vi "总磷通讯.vi"() -> ()   [LabVIEW 2016, in "斯坦道总磷.lvlib"]
uses:
  <vilib>/NI/Modbus Library/API/Wrapper/Create TCP Slave.vi
  <vilib>/Utility/config.llb/Write Key (Boolean).vi
  <vilib>/Utility/config.llb/Write Key (String).vi
  <vilib>/Plasmionique/MB Master/MB_Master/MB_Master.lvclass
  <vilib>/NI/Modbus Library/API/slave/Modbus Slave.lvclass
  <vilib>/Utility/config.llb/NI_LVConfig.lvlib
  <vilib>/Plasmionique/MB Master/MB Master.lvlib
  <vilib>/NI/Modbus Library/API/Wrapper/API Main.lvlib
panel:
  out "总氮测量数据区":u16[](array[numeric])
  out "总氮状态告警区":u16[](array[numeric])
  out "总磷状态告警区":u16[](array[numeric])
  out "总磷测量数据区":u16[](array[numeric])
  out "序列号":string
  out "状态告警区":T1
  out "测量数据区":T2 {"单位" items=["ug/L", "mg/L", "ppm", "mg/m3", "cm", "ppb", "ug/m3", "%", "nmol/mol", "umol/mol", "MPN/L", "MPN/100ml", "ng/m3", "NTU", "无量纲", "ms/cm", "us/cm", "℃", "mV", "万个/L"]}
  out "status":bool
  out "关键参数区":T3
  in  "读关键参数区":bool
  in  "读状态告警区":bool
  in  "读测量数据区":bool
  in  "站号":u16(ring) items=["总磷"=1, "氨氮"=3]
  in  "停止":bool
  in  "启动":bool
  in  "控制命令":u16(ring) items=["启动测量"=1, "标样核查"=2, "零点核查"=3, "跨度核查"=4, "空白测试"=5, "平行样测试"=6, "加标回收"=7, "空白校准"=8, "标样校准"=9, "初始化（清洗）"=10, "停止测试"=11, "仪器重启"=12, "校时"=13, "模式设置"=14, "测量间隔设置"=15]
  in  "控制命令参数":u16[](array[numeric]) format="%04xH"
  in  "VISA Resource":refnum<visa-resource-name>
  in  "启用模块":bool
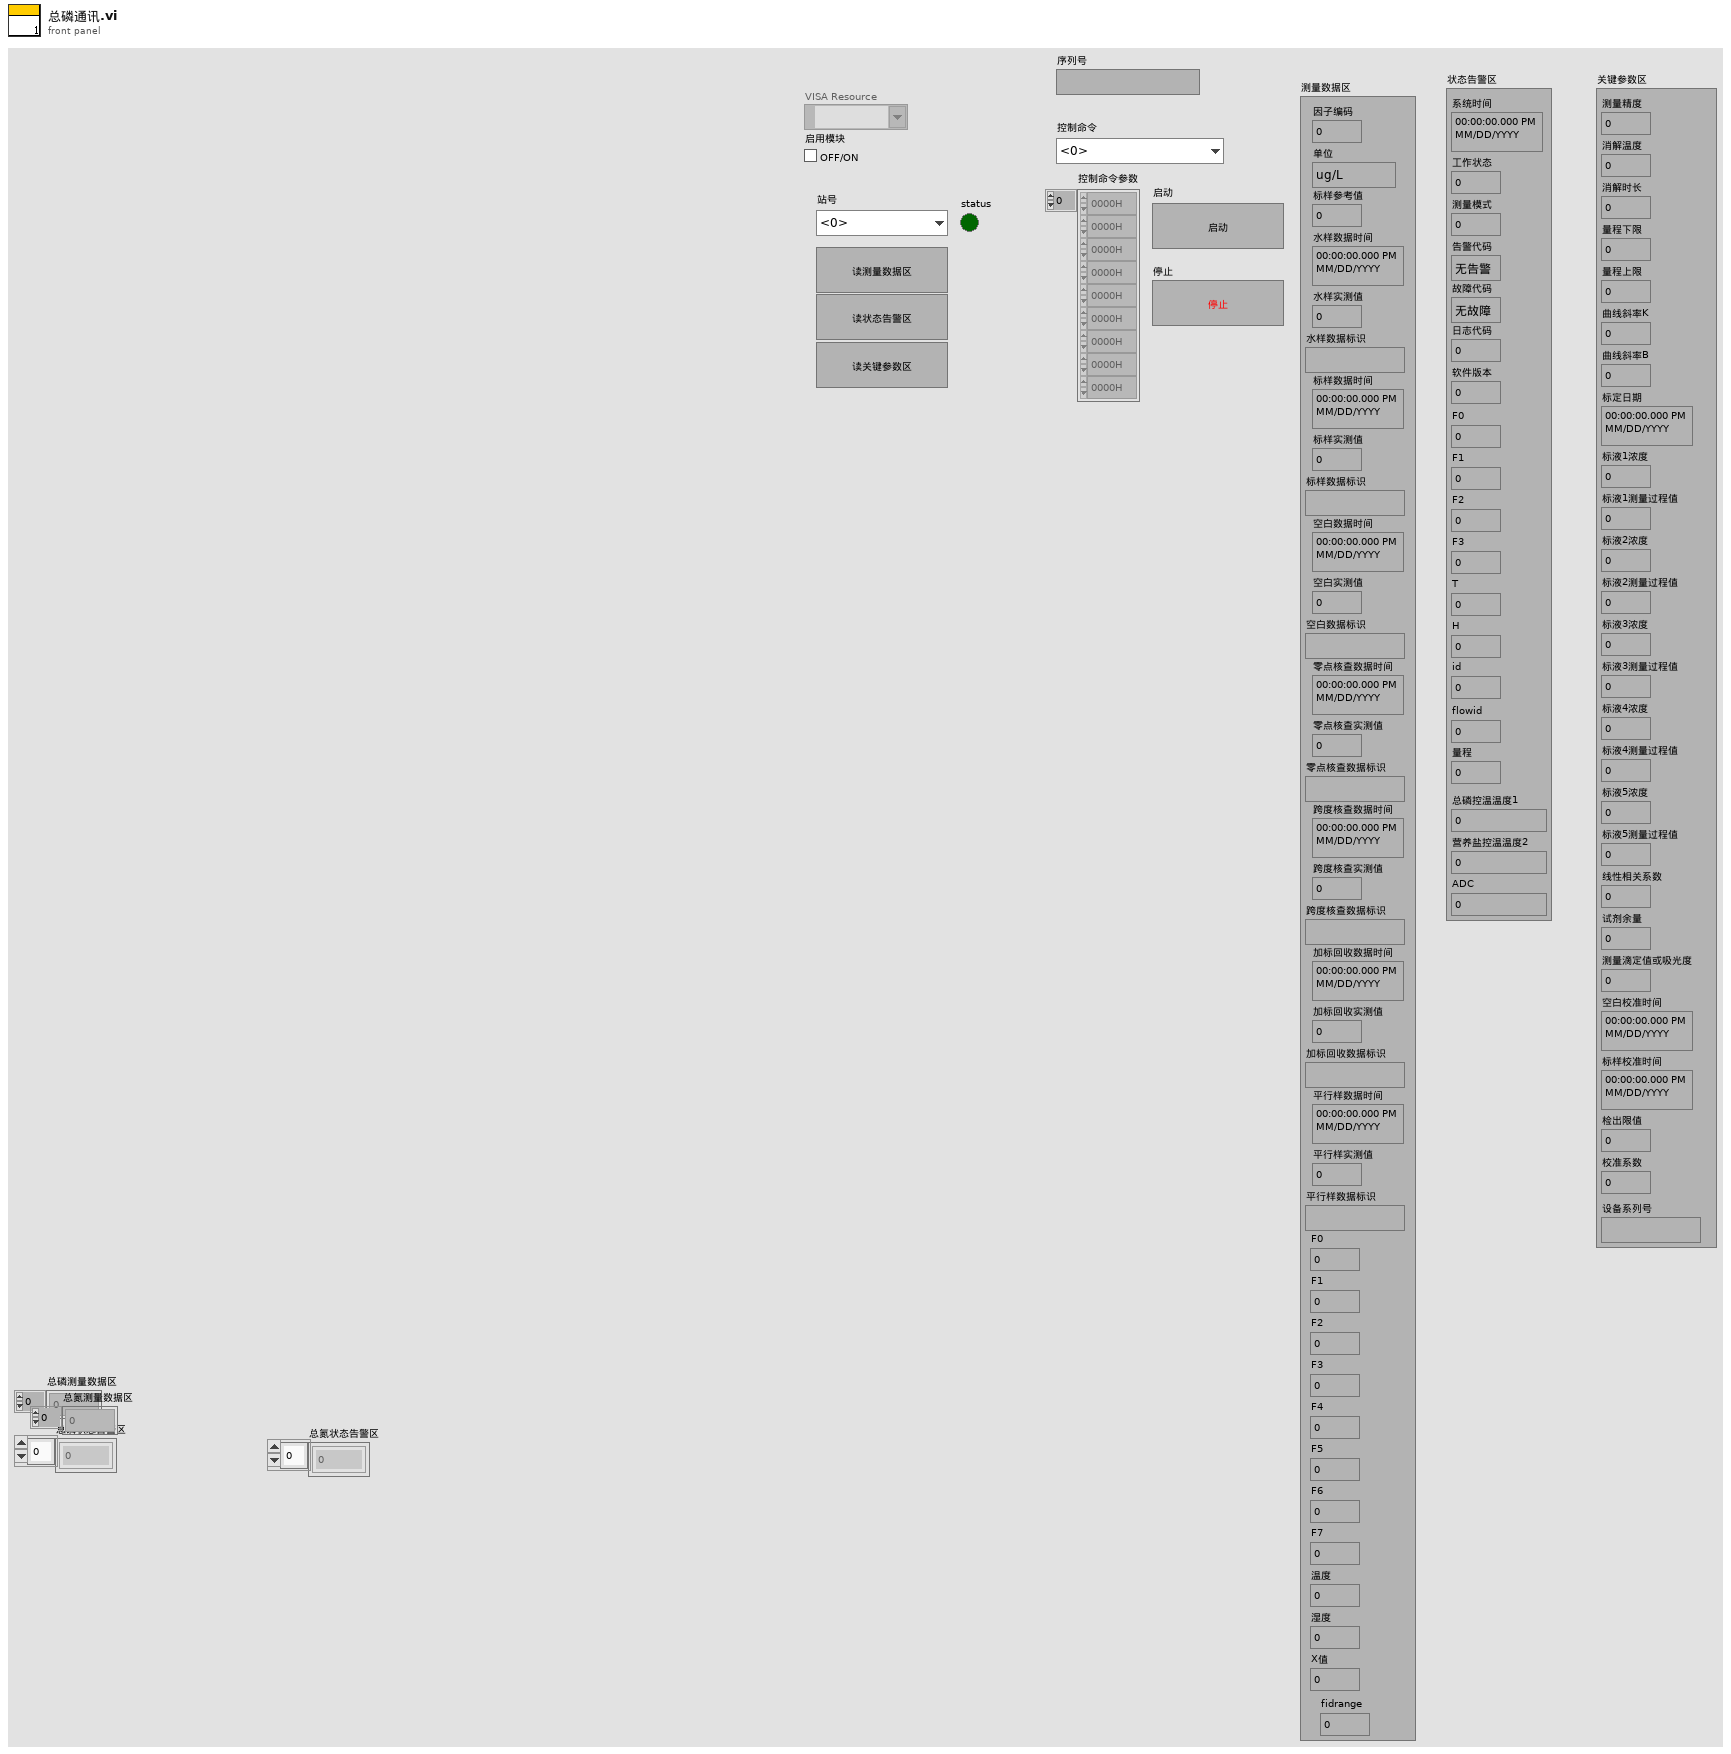
[diagram p1: front panel]
types:
  T1 = cluster{"系统时间":timestamp, "工作状态":u16, "测量模式":u16, "告警代码":enum16{"无告警", "缺试剂告警", "缺水样告警", "缺蒸馏水告警", "缺标液告警", "仪表漏液告警", "标定异常告警", "超量程告警", "加热异常", "低试剂预警", "超上限告警", "超下限告警", "仪表内部其他异常", "滴定异常告警", "电极异常告警", "量程切换告警", "参数设置告警", "PH电极电位异常", "电导率电极异常", "浊度光度异常", "溶解氧电极异常", "溶解氧光强异常", "温度异常告警", "PH异常告警", "溶解氧异常告警", "电导率异常告警", "浊度异常告警", "叶绿素异常告警", "藻密度异常告警", "蓝绿藻异常告警", "ORP异常告警", "氨氮异常告警", "清洁刷异常告警", "SD卡异常告警", "蓝牙异常告警", "Wifi异常告警", "流程异常告警"}, "故障代码":enum16{"无故障", "电机故障", "温度故障", "通讯故障", "滴定故障"}, "日志代码":u16, "软件版本":u16, "F0":sgl, "F1":sgl, "F2":sgl, "F3":sgl, "T":sgl, "H":sgl, "id":u16, "flowid":u16, "量程":u16, "总磷控温温度1":sgl, "营养盐控温温度2":sgl, "ADC":sgl}
  T2 = cluster{"因子编码":u32, "单位":u16, "标样参考值":sgl, "水样数据时间":timestamp, "水样实测值":sgl, "水样数据标识":string, "标样数据时间":timestamp, "标样实测值":sgl, "标样数据标识":string, "空白数据时间":timestamp, "空白实测值":sgl, "空白数据标识":string, "零点核查数据时间":timestamp, "零点核查实测值":sgl, "零点核查数据标识":string, "跨度核查数据时间":timestamp, "跨度核查实测值":sgl, "跨度核查数据标识":string, "加标回收数据时间":timestamp, "加标回收实测值":sgl, "加标回收数据标识":string, "平行样数据时间":timestamp, "平行样实测值":sgl, "平行样数据标识":string, "F0":sgl, "F1":sgl, "F2":sgl, "F3":sgl, "F4":sgl, "F5":sgl, "F6":sgl, "F7":sgl, "温度":sgl, "湿度":sgl, "X值":sgl, "fidrange":u16}
  T3 = cluster{"测量精度":u16, "消解温度":u16, "消解时长":u16, "量程下限":sgl, "量程上限":sgl, "曲线斜率K":sgl, "曲线斜率B":sgl, "标定日期":timestamp, "标液1浓度":sgl, "标液1测量过程值":sgl, "标液2浓度":sgl, "标液2测量过程值":sgl, "标液3浓度":sgl, "标液3测量过程值":sgl, "标液4浓度":sgl, "标液4测量过程值":sgl, "标液5浓度":sgl, "标液5测量过程值":sgl, "线性相关系数":sgl, "试剂余量":u32, "测量滴定值或吸光度":sgl, "空白校准时间":timestamp, "标样校准时间":timestamp, "检出限值":sgl, "校准系数":sgl, "设备系列号":string}
  T4 = typedef "NI_LVConfig.lvlib/Config Data RefNum.ctl" = refnum<k1>
  T5 = enum8{"Enabled", "Disabled", "Disabled and Grayed Out"}
  T6 = cluster{"系统时间":timestamp, "工作状态":enum16{"空闲", "水样测试", "标样核查", "零点核查", "跨度核查", "空白测试", "平行样测试", "加标回收", "空白校准", "标样校准", "初始化（清洗）"}, "测量模式":enum16{"待机", "连续模式", "周期模式", "定点模式", "受控模式", "手动模式"}, "告警代码":enum16{"无告警", "缺试剂告警", "缺水样告警", "缺蒸馏水告警", "缺标液告警", "仪表漏液告警", "标定异常告警", "超量程告警", "加热异常", "低试剂预警", "超上限告警", "超下限告警", "仪表内部其他异常", "滴定异常告警", "电极异常告警", "量程切换告警", "参数设置告警", "PH电极电位异常", "电导率电极异常", "浊度光度异常", "溶解氧电极异常", "溶解氧光强异常", "温度异常告警", "PH异常告警", "溶解氧异常告警", "电导率异常告警", "浊度异常告警", "叶绿素异常告警", "藻密度异常告警", "蓝绿藻异常告警", "ORP异常告警", "氨氮异常告警", "清洁刷异常告警", "SD卡异常告警", "蓝牙异常告警", "Wifi异常告警", "流程异常告警"}, "故障代码":enum16{"无故障", "电机故障", "温度故障", "通讯故障", "滴定故障"}, "日志代码":u16, "软件版本":u16, "F0":sgl, "F1":sgl, "F2":sgl, "F3":sgl, "T":sgl, "H":sgl, "id":u16, "flowid":u16, "量程":u16, "总磷控温温度1":sgl, "营养盐控温温度2":sgl, "ADC":sgl}
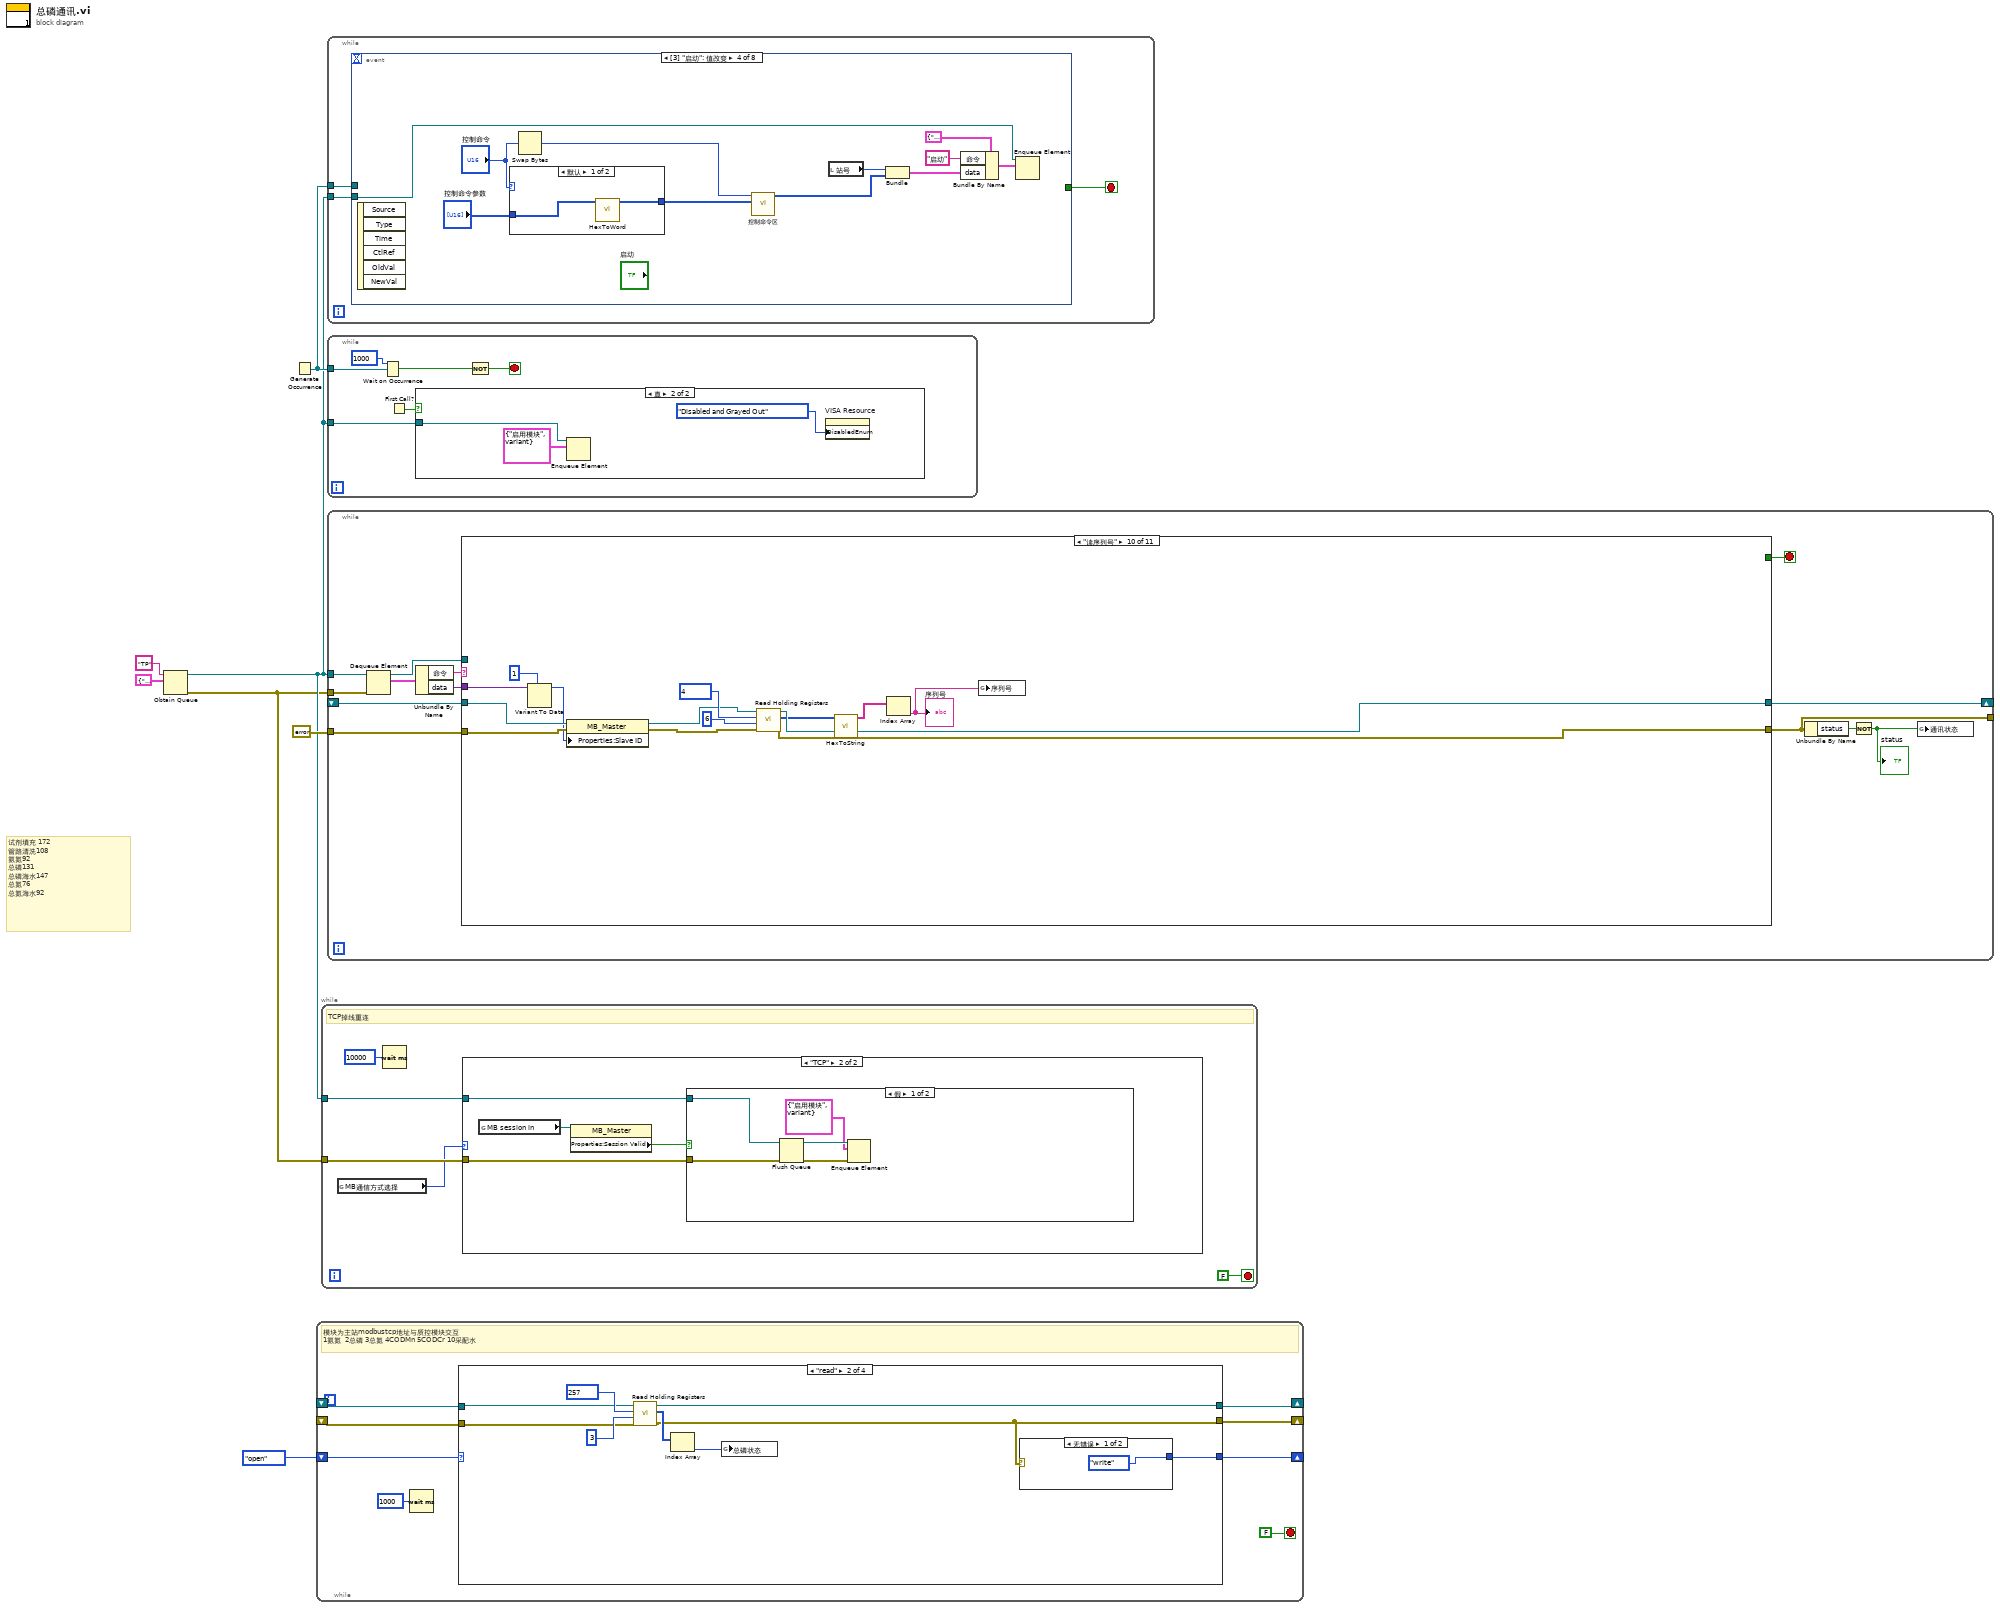
[diagram p0: block diagram]
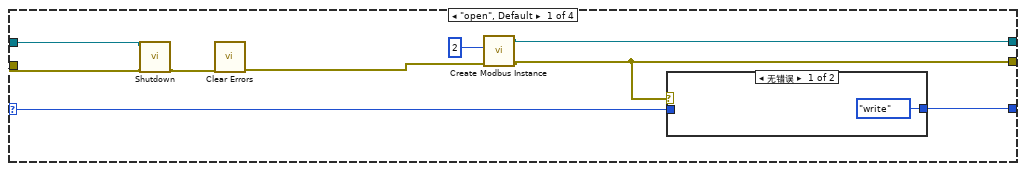
[diagram p4: hidden frame]
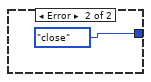
[diagram p6: hidden frame]
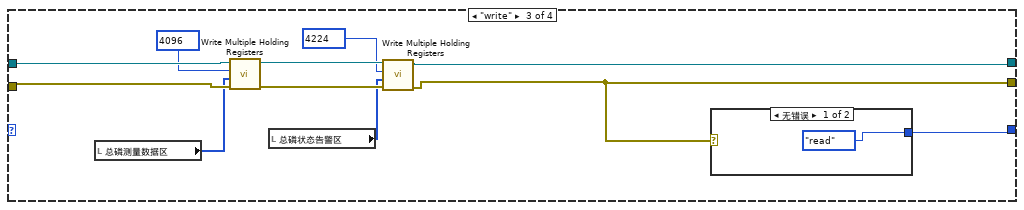
[diagram p7: hidden frame]
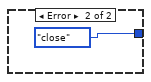
[diagram p8: hidden frame]
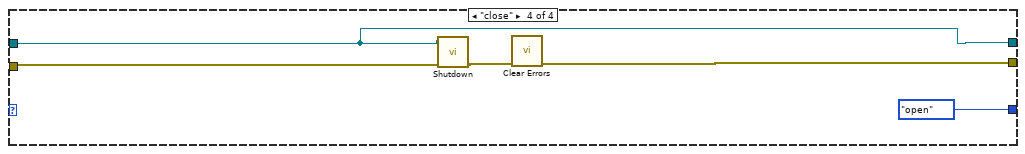
[diagram p9: hidden frame]
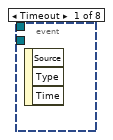
[diagram p11: hidden frame]
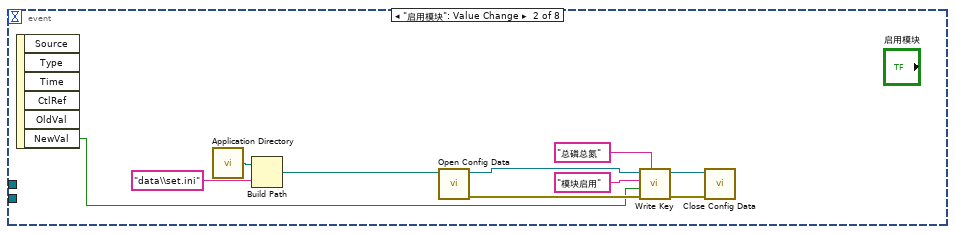
[diagram p12: hidden frame]
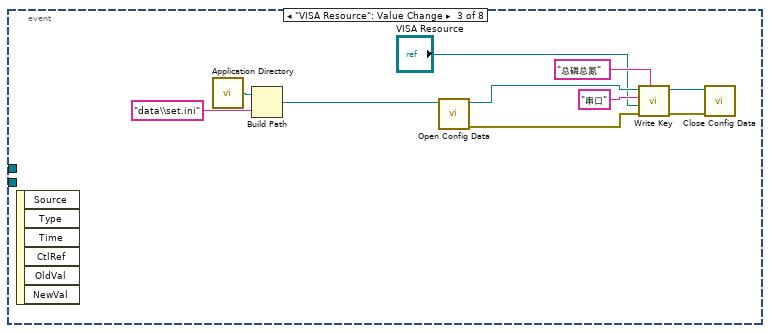
[diagram p13: hidden frame]
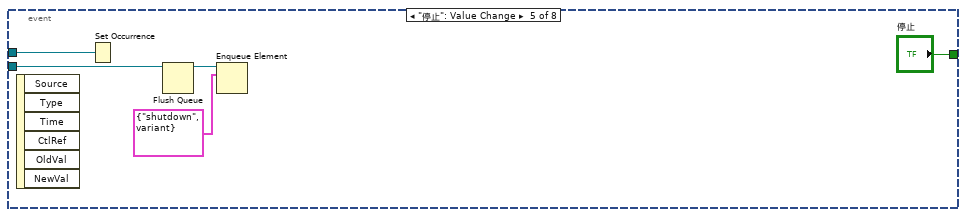
[diagram p15: hidden frame]
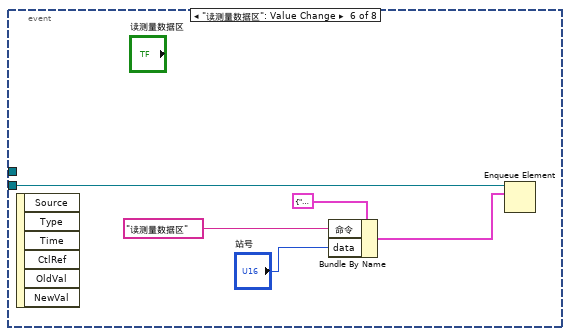
[diagram p16: hidden frame]
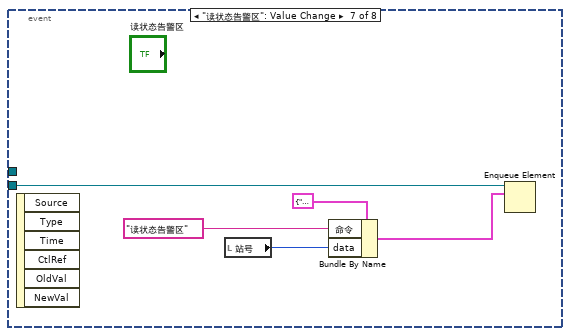
[diagram p17: hidden frame]
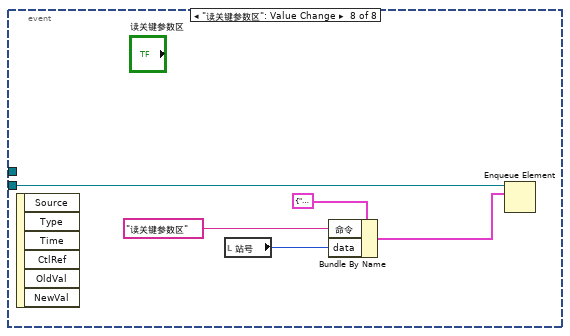
[diagram p18: hidden frame]
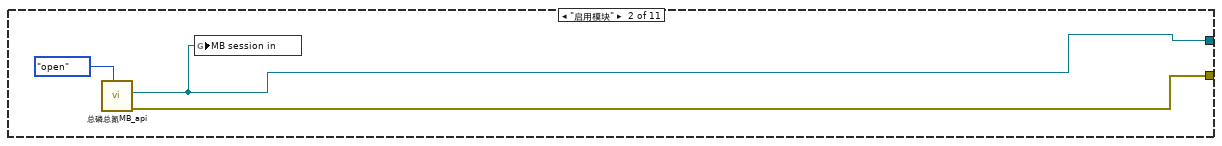
[diagram p20: hidden frame]
diagram:
  # "试剂填充 172 \n管路清洗108\n氨氮92\n总磷131\n总磷海水147\n总氮76\n总氮海水92"
  n1 = Obtain Queue(name (unnamed)="TP" ("名称（未命名）"), element data type=cluster{"命令":string, "data":variant} {"命令"="", "data"=variant}) -> (queue out=w2:refnum<queue>, error out=w1:errorcluster)  [unwired: 3 in, 1 out]
  n2 = Generate Occurrence() -> (w4:refnum<k4>)
  n3 = while {
    shift-right: [w13] -> _
    shift-left: _ -> [w15]
    shift-right: [w12] -> _
    shift-left: _ -> [w14]
    shift-right: [w9] -> _
    shift-left: enum16{"open", "read", "write", "close"}."open" -> [w10]
    stop <- FALSE stop-if-true
    # "模块为主站modbustcp地址与质控模块交互\n1氨氮  2总磷 3总氮 4CODMn 5CODCr 10采配水"
    n4 = Wait (ms)(milliseconds to wait=u32 1000 ("等待时间（毫秒）")) -> ()  [unwired: 1 out]
    n5 = case shown="\"read\"" w10 {
      selector: w10 -> [w24 _ _ _]
      tunnel: w15 -> [w18 w31 w47 w53]
      tunnel: w14 -> [w17 w30 w46 w52]
      tunnel: [w21 w29 w42 w53] -> w13
      tunnel: [w20 w28 w41 w55] -> w12
      tunnel: [w23 w35 w48 enum16{"open", "read", "write", "close"}."open"] -> w9
      frame "open", Default {
        n6 = call-dynamic "Shutdown.vi"("error in"=w17, "Modbus slave in"=w18) -> ("error out"=w16:errorcluster)  [unwired: 9 in]
        n7 = call <vilib>:"Clear Errors.vi"("error in (no error)"=w16) -> ("error out"=w19:errorcluster)  [unwired: 5 in, 1 out]
        n8 = call-poly <vilib>:"Create Modbus Instance.vi"("error in"=w19, "port (502)"=u16 2) -> ("error out"=w20:errorcluster, "TCP slave instance"=w21:refnum<class "Modbus Slave.lvclass">)  [unwired: 8 in]
        n9 = case shown="无错误" w20 {
          tunnel: w24 -> [_ w26]
          tunnel: [enum16{"open", "read", "write", "close"}."write" w26] -> w23
          frame No Error {
          }
          frame Error {
          }
        }
      }
      frame "read" {
        n10 = call-dynamic <vilib>:"Read Holding Registers.vi"("error in"=w30, "number of inputs"=u16 3, "starting address"=u16 257, "Modbus slave in"=w31) -> ("error out"=w28:errorcluster, "register values"=w32:u16[], "Modbus slave out"=w29:refnum<class "Modbus Slave.lvclass">)  [unwired: 5 in]
        n11 = Index Array(array=w32) -> (element=w27:u16)  [unwired: 1 in]
        n12 = global write "VAR总磷全局变量.vi" "总磷状态"(w27) -> ()
        n13 = case shown="无错误" w28 {
          tunnel: [enum16{"open", "read", "write", "close"}."write" enum16{"open", "read", "write", "close"}."close"] -> w35
          frame No Error {
          }
          frame Error {
          }
        }
      }
      frame "write" {
        n14 = local read "总磷测量数据区"() -> (w40:u16[])
        n15 = call-dynamic "Write Multiple Holding Registers.vi"("error in"=w46, "registers to write"=w40, "starting address"=u16 4096, "Modbus slave in"=w47) -> ("error out"=w43:errorcluster, "Modbus slave out"=w44:refnum<class "Modbus Slave.lvclass">)  [unwired: 6 in]
        n16 = local read "总磷状态告警区"() -> (w38:u16[])
        n17 = call-dynamic "Write Multiple Holding Registers.vi"("error in"=w43, "registers to write"=w38, "starting address"=u16 4224, "Modbus slave in"=w44) -> ("error out"=w41:errorcluster, "Modbus slave out"=w42:refnum<class "Modbus Slave.lvclass">)  [unwired: 6 in]
        n18 = case shown="无错误" w41 {
          tunnel: [enum16{"open", "read", "write", "close"}."read" enum16{"open", "read", "write", "close"}."close"] -> w48
          frame No Error {
          }
          frame Error {
          }
        }
      }
      frame "close" {
        n19 = call-dynamic "Shutdown.vi"("error in"=w52, "Modbus slave in"=w53) -> ("error out"=w51:errorcluster)  [unwired: 9 in]
        n20 = call <vilib>:"Clear Errors.vi"("error in (no error)"=w51) -> ("error out"=w55:errorcluster)  [unwired: 5 in, 1 out]
      }
    }
  }
  n21 = while "While循环" {
    tunnel: w2 -> [w58]
    tunnel: w1 -> [w57]
    stop <- FALSE stop-if-true
    # "TCP掉线重连"
    n22 = global read "总磷断电保存全局变量.vi" "MB通信方式选择"() -> (w56:enum16{"串口", "TCP"})
    n23 = Wait (ms)(milliseconds to wait=u32 10000 ("等待时间（毫秒）")) -> ()  [unwired: 1 out]
    n24 = case shown="\"TCP\"" w56 {
      tunnel: w58 -> [_ w63]
      tunnel: w57 -> [_ w62]
      frame "串口", Default {
      }
      frame "TCP" {
        n25 = global read "VAR总磷全局变量.vi" "MB session in"() -> (w61:refnum<class "MB_Master.lvclass">)
        n26 = property class="MB_Master"(reference=w61) -> ("Properties:Session Valid"=w64:bool)  [unwired: 1 in, 2 out]
        n27 = case shown="假" w64 {
          tunnel: w63 -> [w67 _]
          tunnel: w62 -> [w66 _]
          frame False {
            n28 = Flush Queue(queue=w67, error in (no error)=w66) -> (queue out=w69:refnum<queue>, error out=w68:errorcluster)  [unwired: 1 out]
            n29 = Enqueue Element(queue=w69, element=cluster{"命令":string, "data":variant} {"命令"="启用模块", "data"=variant} ("元素"), error in (no error)=w68) -> ()  [unwired: 1 in, 3 out]
          }
          frame True {
          }
        }
      }
    }
  }
  n30 = while {
    tunnel: w2 -> [w72]
    tunnel: w4 -> [w70]
    stop <- w71 stop-if-true
    n31 = event shown="[3] \"启动\": 值改变" {
      selector: _ -> [_ _ _ _ _ _ _ _]
      dyn-events: _ -> [_ _ _ _ _ _ _ _]
      timeout: _ -> [_ _ _ _ _ _ _ _]
      tunnel: w72 -> [_ _ _ w103 w110 w116 w121 w126]
      tunnel: [_ _ _ _ "停止" _ _ _] -> w71
      tunnel: w70 -> [_ _ _ _ w107 _ _ _]
      event Timeout {
        n32 = event-data() -> ()  [unwired: 1 in, 3 out]
      }
      event "启用模块": Value Change {
        n33 = event-data() -> ("NewVal"=w73:bool)  [unwired: 1 in, 5 out]
        n34 = call <vilib>:"Application Directory.vi"() -> ("Application Directory"=w75:path)
        n35 = Build Path(base path=w75, name or relative path="data\\set.ini" ("名称或相对路径")) -> (appended path=w76:path)
        n36 = call <vilib>:"Open Config Data.vi"("configuration file path"=w76) -> ("error out"=w82:errorcluster, "refnum"=w81:T4)  [unwired: 8 in, 1 out]
        n37 = call-poly <vilib>:"Write Key.vi"("section"="总磷总氮", "error in (no error)"=w82, "value"=w73, "key"="模块启用", "refnum"=w81) -> ("error out"=w78:errorcluster, "refnum out"=w74:T4)  [unwired: 4 in, 1 out]
        n38 = call <vilib>:"Close Config Data.vi"("error in (no error)"=w78, "refnum"=w74) -> ()  [unwired: 8 in, 2 out]
      }
      event "VISA Resource": Value Change {
        n39 = event-data() -> ()  [unwired: 1 in, 6 out]
        n40 = call <vilib>:"Application Directory.vi"() -> ("Application Directory"=w85:path)
        n41 = Build Path(base path=w85, name or relative path="data\\set.ini" ("名称或相对路径")) -> (appended path=w86:path)
        n42 = call <vilib>:"Open Config Data.vi"("configuration file path"=w86) -> ("error out"=w92:errorcluster, "refnum"=w91:T4)  [unwired: 8 in, 1 out]
        n43 = call-poly <vilib>:"Write Key.vi"("section"="总磷总氮", "error in (no error)"=w92, "value"="VISA Resource", "key"="串口", "refnum"=w91) -> ("error out"=w88:errorcluster, "refnum out"=w84:T4)  [unwired: 4 in, 1 out]
        n44 = call <vilib>:"Close Config Data.vi"("error in (no error)"=w88, "refnum"=w84) -> ()  [unwired: 8 in, 2 out]
      }
      event "启动": Value Change {
        n45 = event-data() -> ()  [unwired: 1 in, 6 out]
        n46 = case shown="默认" "控制命令" {
          tunnel: "控制命令参数" -> [w105 w106]
          tunnel: [w104 w106] -> w93
          frame Default {
            n47 = call "HexToWord.vi"("数组"=w105) -> ("WORD"=w104:u16[])  [unwired: 10 in]
          }
          frame 13 {
          }
        }
        n48 = Swap Bytes(anything="控制命令") -> (byte swapped=w96:u16)
        n49 = call "控制命令区.vi"("控制命令参数"=w93, "控制命令"=w96) -> ("控制命令"=w99:u16[])  [unwired: 9 in]
        n50 = local read "站号"() -> (w98:u16)
        n51 = Bundle("站号"=w98, "控制命令"=w99) -> (w97:cluster{"站号":u16, "控制命令":u16[]})  [unwired: 1 in]
        n52 = Bundle By Name(cluster=cluster{"命令":string, "data":variant} {"命令"="", "data"=variant} ("元素"), "命令"="启动", "data"=w97) -> (w101:cluster{"命令":string, "data":variant})
        n53 = Enqueue Element(queue=w103, element=w101) -> ()  [unwired: 2 in, 3 out]
      }
      event "停止": Value Change {
        n54 = event-data() -> ()  [unwired: 1 in, 6 out]
        n55 = Set Occurrence(w107) -> ()
        n56 = Flush Queue(queue=w110) -> (queue out=w109:refnum<queue>)  [unwired: 1 in, 2 out]
        n57 = Enqueue Element(queue=w109, element=cluster{"命令":string, "data":variant} {"命令"="shutdown", "data"=variant} ("元素")) -> ()  [unwired: 2 in, 3 out]
      }
      event "读测量数据区": Value Change {
        n58 = event-data() -> ()  [unwired: 1 in, 6 out]
        n59 = Bundle By Name(cluster=cluster{"命令":string, "data":variant} {"命令"="", "data"=variant} ("元素"), "命令"="读测量数据区", "data"="站号") -> (w114:cluster{"命令":string, "data":variant})
        n60 = Enqueue Element(queue=w116, element=w114) -> ()  [unwired: 2 in, 3 out]
      }
      event "读状态告警区": Value Change {
        n61 = event-data() -> ()  [unwired: 1 in, 6 out]
        n62 = local read "站号"() -> (w117:u16)
        n63 = Bundle By Name(cluster=cluster{"命令":string, "data":variant} {"命令"="", "data"=variant} ("元素"), "命令"="读状态告警区", "data"=w117) -> (w119:cluster{"命令":string, "data":variant})
        n64 = Enqueue Element(queue=w121, element=w119) -> ()  [unwired: 2 in, 3 out]
      }
      event "读关键参数区": Value Change {
        n65 = event-data() -> ()  [unwired: 1 in, 6 out]
        n66 = local read "站号"() -> (w122:u16)
        n67 = Bundle By Name(cluster=cluster{"命令":string, "data":variant} {"命令"="", "data"=variant} ("元素"), "命令"="读关键参数区", "data"=w122) -> (w124:cluster{"命令":string, "data":variant})
        n68 = Enqueue Element(queue=w126, element=w124) -> ()  [unwired: 2 in, 3 out]
      }
    }
  }
  n69 = while {
    tunnel: w4 -> [w132]
    tunnel: w2 -> [w128]
    stop <- w129 stop-if-true
    n70 = Wait on Occurrence(2:w132, 3:1000 ("毫秒超时(-1)")) -> (0:w130:bool)  [unwired: 1 in]
    n71 = First Call?() -> (First Call?: T/F=w127:bool)
    n72 = case shown="真" w127 {
      tunnel: w128 -> [_ w134]
      frame False {
      }
      frame True {
        n73 = Enqueue Element(queue=w134, element=cluster{"命令":string, "data":variant} {"命令"="启用模块", "data"=variant} ("元素")) -> ()  [unwired: 2 in, 3 out]
        n74 = property on="VISA Resource" class="VISAName"("DisabledEnum"=T5."Disabled and Grayed Out" ("禁用")) -> ()  [unwired: 2 in, 2 out]
      }
    }
    n75 = Not(x=w130) -> (.not. x?=w129:bool)
  }
  n76 = while {
    tunnel: w2 -> [w148]
    tunnel: w1 -> [w147]
    shift-right: [w145] -> _
    shift-left: _ -> [w144]
    tunnel: errorcluster {"status"=FALSE, "code"=0, "source"=""} ("error out") -> [w143]
    tunnel: [w138] -> _
    stop <- w146 stop-if-true
    n77 = Dequeue Element(queue=w148, error in (no error)=w147) -> (queue out=w139:refnum<queue>, element=w141:cluster{"命令":string, "data":variant})  [unwired: 1 in, 2 out]
    n78 = Unbundle By Name(w141) -> ("命令"=w142:string, "data"=w140:variant)
    n79 = case shown="\"读序列号\"" w142 {
      tunnel: w140 -> [_ _ _ w167 w178 w195 w205 w219 w237 w251 _]
      tunnel: w139 -> [_ _ _ _ _ _ _ _ _ _ w264]
      tunnel: [_ _ _ _ _ _ _ _ _ _ TRUE] -> w146
      tunnel: [w149 w152 w154 w170 w181 w197 w209 w228 w244 w258 w260] -> w145
      tunnel: [w150 w151 w155 w169 w180 w196 w210 w218 w245 w259 w261] -> w138
      tunnel: w144 -> [w149 _ w154 w166 w177 w194 w204 w222 w240 w254 w260]
      tunnel: w143 -> [w150 _ w157 w163 w174 w191 w202 w223 w241 w255 w262]
      frame Default {
      }
      frame "启用模块" {
        n80 = call "总磷总氮MB_api.vi"("STEP"=enum16{"open", "read", "write", "close"}."open") -> ("error out"=w151:errorcluster, "MB session out"=w152:refnum<class "MB_Master.lvclass">)  [unwired: 8 in, 1 out]
        n81 = global write "VAR总磷全局变量.vi" "MB session in"(w152) -> ()
      }
      frame "停用模块" {
        n82 = call-dynamic "Close Session.vi"("error in (no error)"=w157, "MB session in"=w154) -> ("error out"=w156:errorcluster)  [unwired: 9 in]
        n83 = call <vilib>:"Clear Errors.vi"("error in (no error)"=w156) -> ("error out"=w155:errorcluster)  [unwired: 5 in, 1 out]
      }
      frame "启动" {
        n84 = Variant To Data(type=cluster{"站号":u16, "控制命令":u16[]} {"站号"=0, "控制命令"=[]} ("输出簇"), Variant=w167) -> (data=w161:cluster{"站号":u16, "控制命令":u16[]})  [unwired: 1 in, 1 out]
        n85 = Unbundle By Name(w161) -> ("站号"=w160:u16, "控制命令"=w158:u16[])
        n86 = property class="MB_Master"(reference=w166, error in=w163, "Properties:Slave ID"=w160) -> (reference out=w165:refnum<class "MB_Master.lvclass">, error out=w164:errorcluster)
        n87 = Index Array(array=w158) -> (element=w159:u16)  [unwired: 1 in]
        n88 = global write "VAR总磷全局变量.vi" "控制命令"(w159) -> ()
        n89 = call <vilib>:"Write Multiple Registers.vi"("error in (no error)"=w164, "values"=w158, "starting address"=u16 4608, "MB session in"=w165) -> ("error out"=w169:errorcluster, "MB session out"=w170:refnum<class "MB_Master.lvclass">)  [unwired: 6 in]
      }
      frame "盲样测试" {
        n90 = Variant To Data(type=0, Variant=w178) -> (data=w171:i32)  [unwired: 1 in, 1 out]
        n91 = case shown="默认" w171 {
          tunnel: [u16[] [] ("values") u16[] [33539, 0] ("values") u16[] [23555, 0] ("values")] -> w173
          frame Default {
          }
          frame 1 {
            # "总磷盲样测试命令"
          }
          frame 3 {
            # "氨氮盲样测试"
          }
        }
        n92 = property class="MB_Master"(reference=w177, error in=w174, "Properties:Slave ID"=w171) -> (reference out=w176:refnum<class "MB_Master.lvclass">, error out=w175:errorcluster)
        n93 = call <vilib>:"Write Multiple Registers.vi"("error in (no error)"=w175, "values"=w173, "starting address"=u16 24592, "MB session in"=w176) -> ("error out"=w180:errorcluster, "MB session out"=w181:refnum<class "MB_Master.lvclass">)  [unwired: 6 in]
      }
      frame "debug" {
        n94 = Variant To Data(type=cluster{"站号":u16, "控制命令":u16[]} {"站号"=0, "控制命令"=[]} ("输出簇"), Variant=w195) -> (data=w189:cluster{"站号":u16, "控制命令":u16[]})  [unwired: 1 in, 1 out]
        n95 = Unbundle By Name(w189) -> ("站号"=w188:u16, "控制命令"=w186:u16[])
        n96 = property class="MB_Master"(reference=w194, error in=w191, "Properties:Slave ID"=w188) -> (reference out=w193:refnum<class "MB_Master.lvclass">, error out=w192:errorcluster)
        n97 = Index Array(array=w186) -> (element=w187:u16)  [unwired: 1 in]
        n98 = global write "VAR总磷全局变量.vi" "控制命令"(w187) -> ()
        n99 = call <vilib>:"Write Multiple Registers.vi"("error in (no error)"=w192, "values"=w186, "starting address"=u16 24594, "MB session in"=w193) -> ("error out"=w196:errorcluster, "MB session out"=w197:refnum<class "MB_Master.lvclass">)  [unwired: 6 in]
      }
      frame "读测量数据区" {
        n100 = Variant To Data(type=u8 1 ("Slave ID"), Variant=w205) -> (data=w200:u8)  [unwired: 1 in, 1 out]
        n101 = property class="MB_Master"(reference=w204, error in=w202, "Properties:Slave ID"=w200) -> (reference out=w203:refnum<class "MB_Master.lvclass">, error out=w201:errorcluster)
        n102 = call <vilib>:"Read Holding Registers.vi"("error in (no error)"=w201, "quantity"=u16 105, "starting address"=u16 4096, "MB session in"=w203) -> ("error out"=w210:errorcluster, "Registers"=w199:u16[], "MB session out"=w209:refnum<class "MB_Master.lvclass">)  [unwired: 5 in]
        n103 = call "测量数据区.vi"("数组"=w199) -> ("测量数据区"=w198:T2)  [unwired: 10 in]
        "测量数据区" <- w198
        n104 = case shown="1" w200 {
          tunnel: w198 -> [_ w211 w213]
          tunnel: w199 -> [_ w212 w214]
          frame 0, Default {
          }
          frame 1 {
            n105 = global write "VAR总磷全局变量.vi" "总磷测量数据区"(w211) -> ()
            "总磷测量数据区" <- w212
          }
          frame 2 {
            n106 = global write "VAR总磷全局变量.vi" "总氮测量数据区"(w213) -> ()
            "总氮测量数据区" <- w214
          }
        }
        n107 = global write "VAR总磷全局变量.vi" "测量数据区"(w198) -> ()
      }
      frame "读状态告警区" {
        n108 = Variant To Data(type=u8 1 ("Slave ID"), Variant=w219) -> (data=w224:u8)  [unwired: 1 in, 1 out]
        n109 = property class="MB_Master"(reference=w222, error in=w223, "Properties:Slave ID"=w224) -> (reference out=w221:refnum<class "MB_Master.lvclass">, error out=w220:errorcluster)
        n110 = call <vilib>:"Read Holding Registers.vi"("error in (no error)"=w220, "quantity"=u16 29, "starting address"=u16 4224, "MB session in"=w221) -> ("error out"=w218:errorcluster, "Registers"=w215:u16[], "MB session out"=w228:refnum<class "MB_Master.lvclass">)  [unwired: 5 in]
        n111 = call "状态告警区.vi"("数组"=w215) -> ("状态告警区"=w216:T6)  [unwired: 10 in]
        "状态告警区" <- w216
        n112 = global write "VAR总磷全局变量.vi" "状态告警区"(w216) -> ()
        n113 = Unbundle By Name(w216) -> ("id"=w217:u16)
        n114 = case shown="0, 默认" w217 {
          tunnel: w216 -> [_ w229 w231]
          tunnel: w215 -> [_ w230 w232]
          frame 0, Default {
          }
          frame 1, 131 {
            n115 = global write "VAR总磷全局变量.vi" "总磷状态告警区"(w229) -> ()
            "总磷状态告警区" <- w230
          }
          frame 2, 76 {
            n116 = global write "VAR总磷全局变量.vi" "总氮状态告警区"(w231) -> ()
            "总氮状态告警区" <- w232
          }
        }
      }
      frame "读关键参数区" {
        n117 = Variant To Data(type=u8 1 ("Slave ID"), Variant=w237) -> (data=w235:u8)  [unwired: 1 in, 1 out]
        n118 = property class="MB_Master"(reference=w240, error in=w241, "Properties:Slave ID"=w235) -> (reference out=w239:refnum<class "MB_Master.lvclass">, error out=w238:errorcluster)
        n119 = call <vilib>:"Read Holding Registers.vi"("error in (no error)"=w238, "quantity"=u16 19, "starting address"=u16 4256, "MB session in"=w239) -> ("error out"=w245:errorcluster, "Registers"=w234:u16[], "MB session out"=w244:refnum<class "MB_Master.lvclass">)  [unwired: 5 in]
        n120 = call "关键参数区.vi"("数组"=w234) -> ("关键参数区"=w233:T3)  [unwired: 10 in]
        "关键参数区" <- w233
        n121 = global write "VAR总磷全局变量.vi" "关键参数区"(w233) -> ()
      }
      frame "读序列号" {
        n122 = Variant To Data(type=u8 1 ("Slave ID"), Variant=w251) -> (data=w249:u8)  [unwired: 1 in, 1 out]
        n123 = property class="MB_Master"(reference=w254, error in=w255, "Properties:Slave ID"=w249) -> (reference out=w253:refnum<class "MB_Master.lvclass">, error out=w252:errorcluster)
        n124 = call <vilib>:"Read Holding Registers.vi"("error in (no error)"=w252, "quantity"=u16 6, "starting address"=u16 4, "MB session in"=w253) -> ("error out"=w259:errorcluster, "Registers"=w248:u16[], "MB session out"=w258:refnum<class "MB_Master.lvclass">)  [unwired: 5 in]
        n125 = call "HexToString.vi"("数组"=w248) -> ("STRING"=w247:string[])  [unwired: 10 in]
        n126 = Index Array(array=w247) -> (element=w246:string)  [unwired: 1 in]
        "序列号" <- w246
        n127 = global write "VAR总磷全局变量.vi" "序列号"(w246) -> ()
      }
      frame "shutdown" {
        n128 = call-dynamic "Close Session.vi"("error in (no error)"=w262, "MB session in"=w260) -> ("error out"=w261:errorcluster)  [unwired: 9 in]
        n129 = Flush Queue(queue=w264) -> (queue out=w263:refnum<queue>)  [unwired: 1 in, 2 out]
        n130 = Release Queue(queue=w263) -> ()  [unwired: 2 in, 3 out]
      }
    }
    n131 = Unbundle By Name(w138) -> ("status"=w137:bool)
    n132 = Not(x=w137) -> (.not. x?=w136:bool)
    "status" <- w136
    n133 = global write "VAR总磷全局变量.vi" "通讯状态"(w136) -> ()
  }
